vi "Main.vi"() -> ()   [LabVIEW 2020, in "MVA Message Mapper.lvlib"]
doc: "This template is for the Queued Message Handler design pattern.\n\nThe Event Handling Loop generates messages based on user interface actions.\n\nThe Message Handling Loop processes messages generated by the Event Handling Loop, or by other messages. The messages are string values, so new messages can be added easily to the Message Cases case structure in the Message Handling Loop. Each message cluster can also provide an optional value for Message Data, which is a variant that can be converted to whatever message-specific data is required."
uses:
  <vilib>/gpm_packages/@cs/Bus-message-mapper/Source/MVA Message Mapper.lvlib
  <vilib>/gpm_packages/@cs/Bus-message-mapper/Source/controls/UI Data.ctl
  <vilib>/gpm_packages/@cs/Bus-message-mapper/Source/controls/Message Map.ctl
  <vilib>/gpm_packages/@cs/Bus-message-mapper/Source/controls/Map Key.ctl
  <vilib>/gpm_packages/@cs/Bus-message-mapper/Source/controls/Datum Endpoint Set.ctl
  <vilib>/gpm_packages/@cs/Bus-message-mapper/Source/controls/Datum Endpoint.ctl
  <vilib>/gpm_packages/@cs/Bus-message-mapper/Source/support/MVA Comms/MVA Comms VI Instance.lvclass
  <vilib>/gpm_packages/@cs/Bus-message-mapper/Source/support/Format Into String Test/Format Into String.lvclass
  C:/Program Files/National Instruments/LabVIEW 2020/vi.lib/gpm_packages/@cs/Bus-message-mapper/Source/support/Traversal Algorithm/Node Test.lvclass
  <vilib>/gpm_packages/@cs/Bus-message-mapper/Source/support/Build Array Test/Build Array.lvclass
  <vilib>/Utility/miscctls.llb/LVMapReplaceAction.ctl
  <vilib>/gpm_packages/@cs/Bus-message-mapper/Source/support/MVA Comms/MVA Comms VI Instance.lvclass/MVA Comms VI Instance.ctl
  <vilib>/gpm_packages/@cs/Bus-message-mapper/Source/support/MVA Comms/Accessors/Read Broadcaster.vi
  <vilib>/gpm_packages/@cs/Bus-message-mapper/Source/support/Message Queue/Enqueue Message (Single).vi
  <vilib>/Utility/error.llb/Error Cluster From Error Code.vi
  <vilib>/ErrorRing/Error Ring.xnode
panel:
  in  "Load Cache":bool
  out "Refresh Progress":u32(slide) scale=-1.0..37.0
  in  "Cancel Generate":bool
  in  "Generate Cache":bool
  in  "Exit":bool
  in  "Tab Control":enum32{"Message View", "Actor View"}(tab)
  in  "Messages":i32(listbox)=-1
  in  "Broadcasters":i32(listbox)=-1
  in  "Receivers":i32(listbox)=-1
  in  "Actor's Receivers":i32(listbox)=-1
  in  "Actor's Broadcasters":i32(listbox)=-1
  in  "Actor List":i32(listbox)=-1
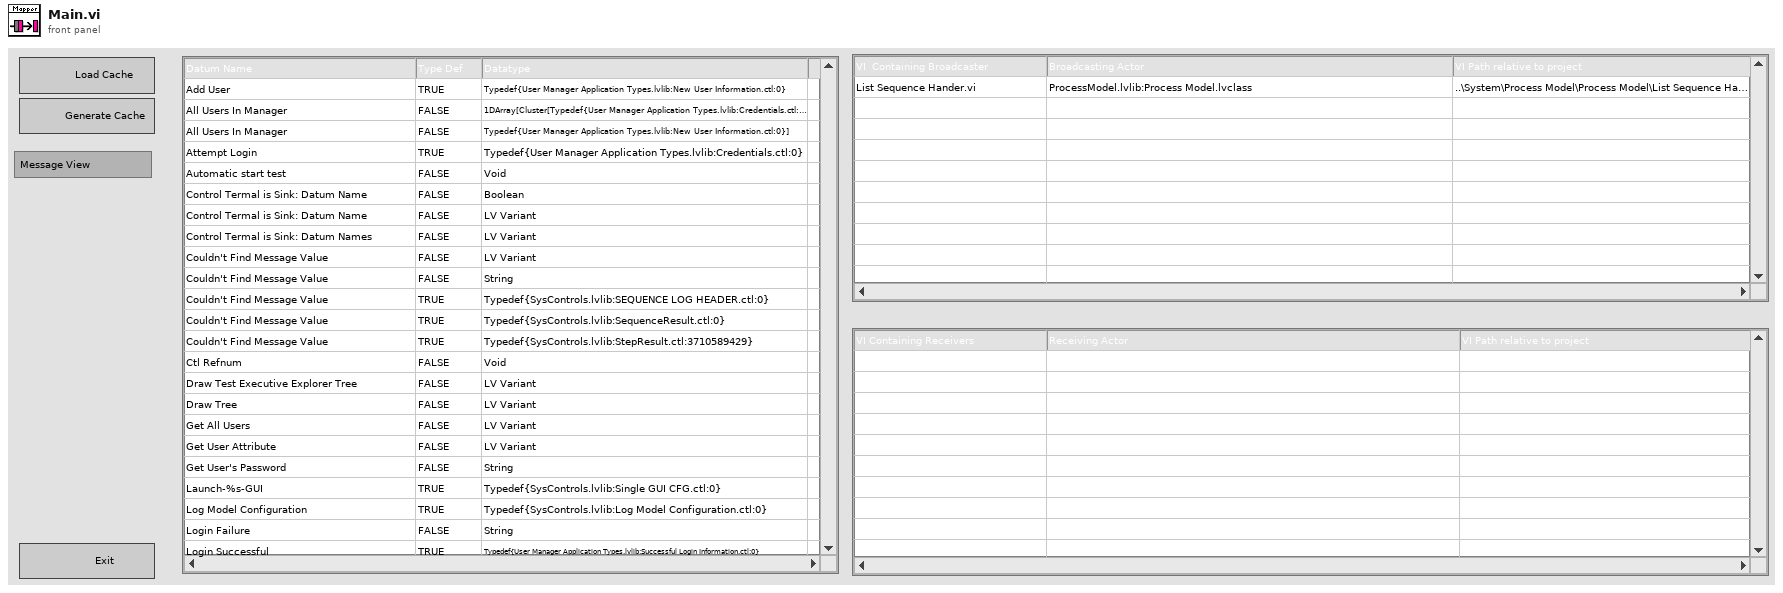
[diagram p1: front panel]
types:
  T1 = typedef "MVA Message Mapper.lvlib/UI Data.ctl" = cluster{"MVA Project Reference":refnum<vi>, "MVA Project Path":path, "Target SubVi Refs":refnum<vi>[], "Targe VI Name":string, "Message View Map":T2, "Broadcaster":bool, "Datum Name Terminal":i32, "Datum Value Terminal":i32, "UI references":cluster{"Message List":refnum<vi>, "Broadcasters":refnum<vi>, "Receivers":refnum<vi>, "Exit Button Ref":refnum<vi>, "Cache Generation Progress":refnum<vi>, "Canced Refresh":refnum<vi>, "Generate Cache":refnum<vi>, "Front Panel":refnum<vi>, "Actor View Receivers":refnum<vi>, "Actor View Broadcasters":refnum<vi>, "Actor View List":refnum<vi>}, "Message Mapper Cache File":path, "MVA Coms VI Instances":refnum<class "MVA Comms VI Instance.lvclass">[], "Cache Generation Marker":u32, "Number of instances":u32, "This VI":refnum<vi>, "Message Map Keys":T3[], "Actor View Map":map{string, cluster{"Datum Broadcasters":T4, "Datum Receivers":T4}}}
  T2 = typedef "MVA Message Mapper.lvlib/Message Map.ctl" = map{T3, cluster{"Datum Broadcasters":T4, "Datum Receivers":T4}}
  T3 = typedef "MVA Message Mapper.lvlib/Map Key.ctl" = cluster{"Datum Name":string, "Value is TypeDef":bool, "Type String":string}
  T4 = typedef "MVA Message Mapper.lvlib/Datum Endpoint Set.ctl" = set{T5}
  T5 = typedef "MVA Message Mapper.lvlib/Datum Endpoint.ctl" = cluster{"Callng VI":path, "Bus VI Name":string, "Source UID":i32, "Sink UID":i32, "Owning Class":string, "Datum Info":T3}
  T6 = typedef "MVA Message Mapper.lvlib/All Message Queues.ctl" = cluster{"UI":refnum<queue>}
  T7 = typedef "LVMapReplaceAction.ctl" = enum32{"Modify Entry only if found", "Add or Modify Entry", "Delete Entry"}
  T8 = enum16{"open", "replace", "create", "open or create", "replace or create", "replace or create with confirmation"}
  T9 = cluster{"VI Name":string, "Owning Actor":string, "Sink UID":string, "Source UID":string}
  T10 = enum32{"Invalid", "Standard", "Closed", "Hidden", "Minimized", "Maximized"}
  T11 = cluster{"Datum Broadcasters":T4, "Datum Receivers":T4}
  T12 = map{string, cluster{"Broadcasters":T4, "Receivers":T4}}
  T13 = map{string, cluster{"Datum Broadcasters":T4, "Datum Receivers":T4}}
  T14 = typedef "LVPoint32TypeDef.ctl" = cluster{"Horizontal":i32, "Vertical":i32}
  T15 = typedef "LVRowAndColumnTypeDef.ctl" = cluster{"Row":i32, "Column":i32}
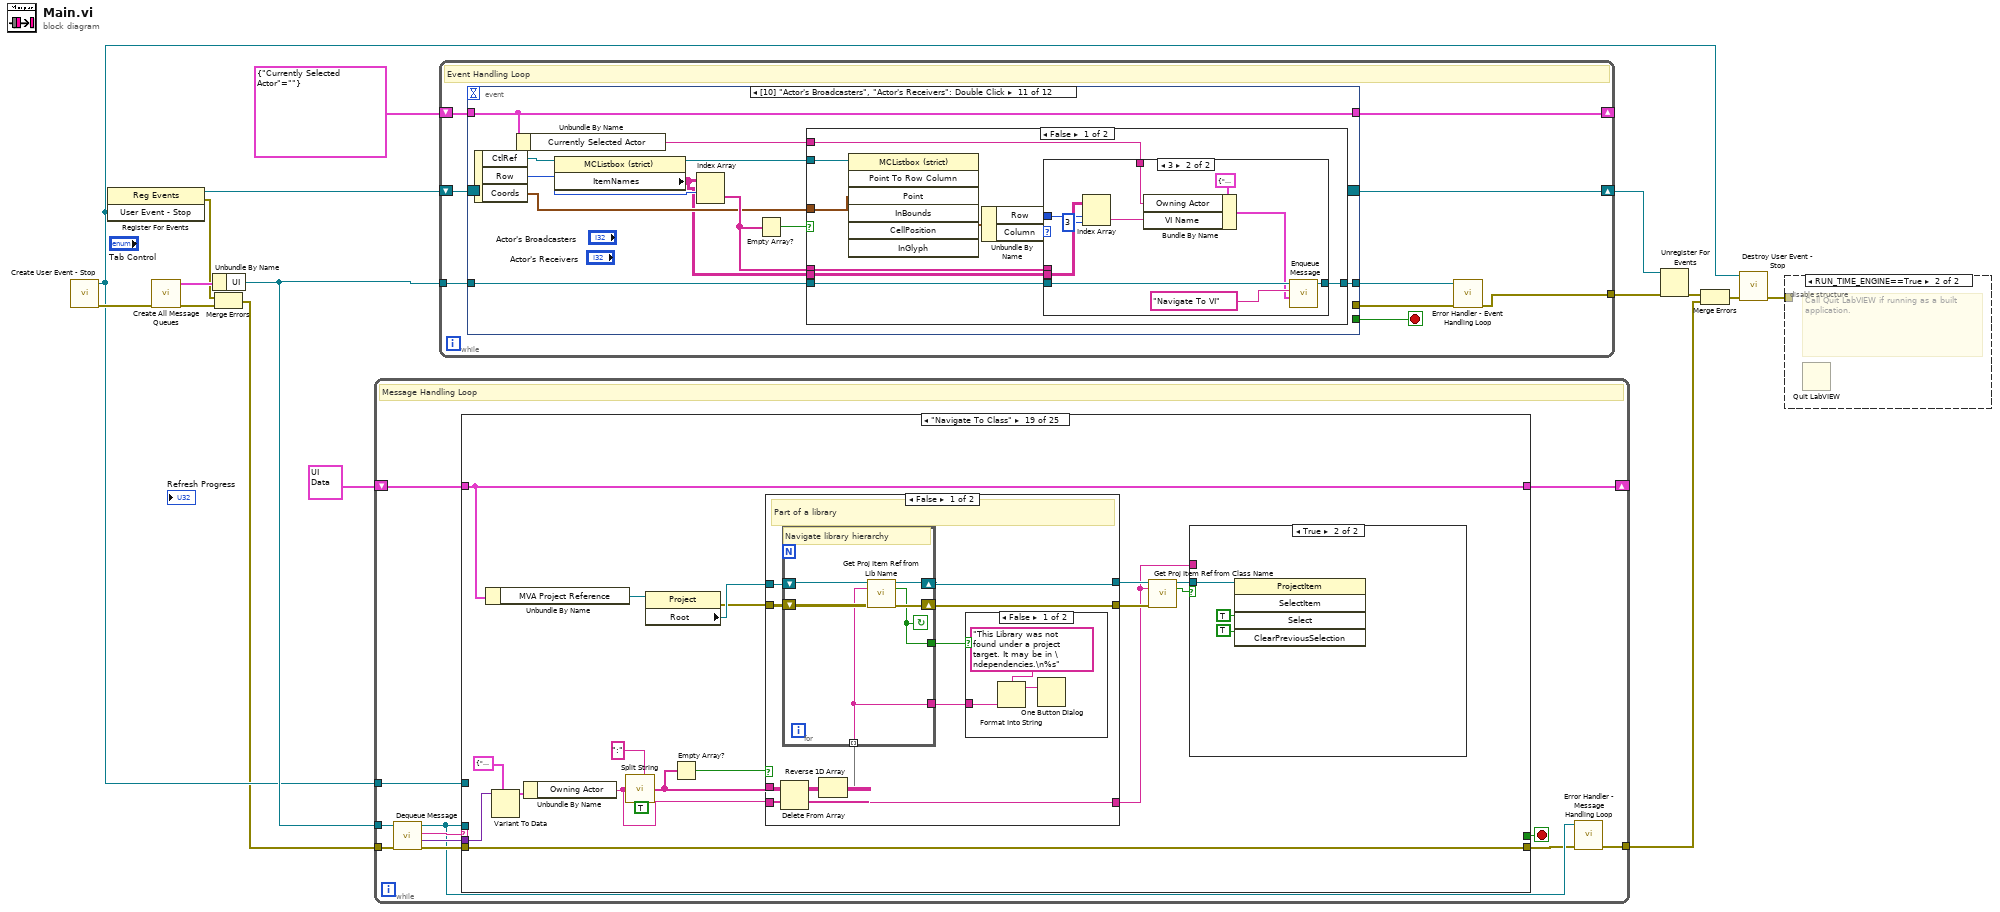
[diagram p0: block diagram]
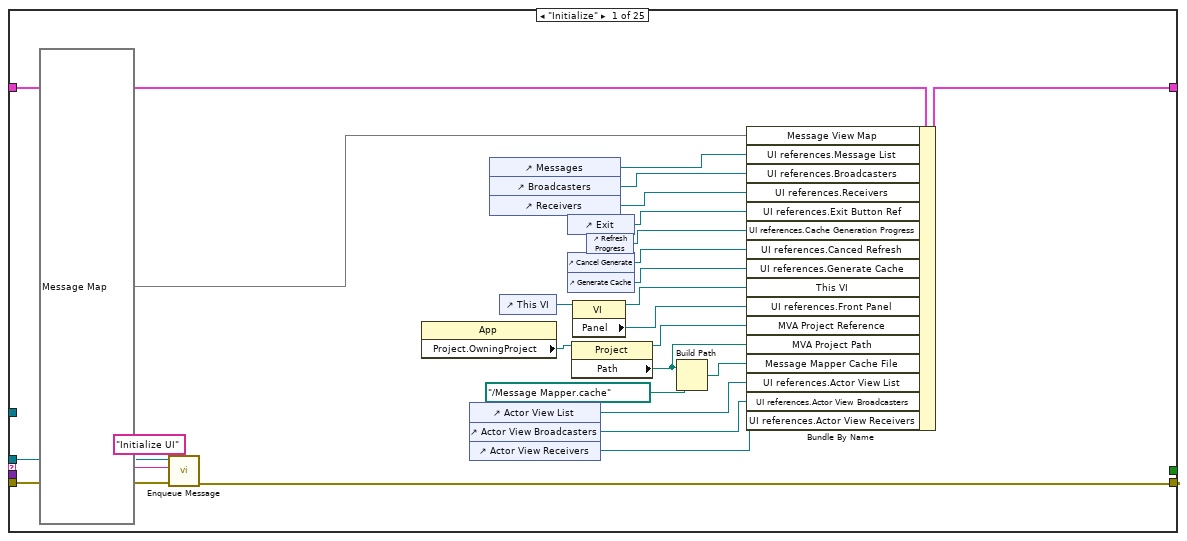
[diagram p2: hidden frame]
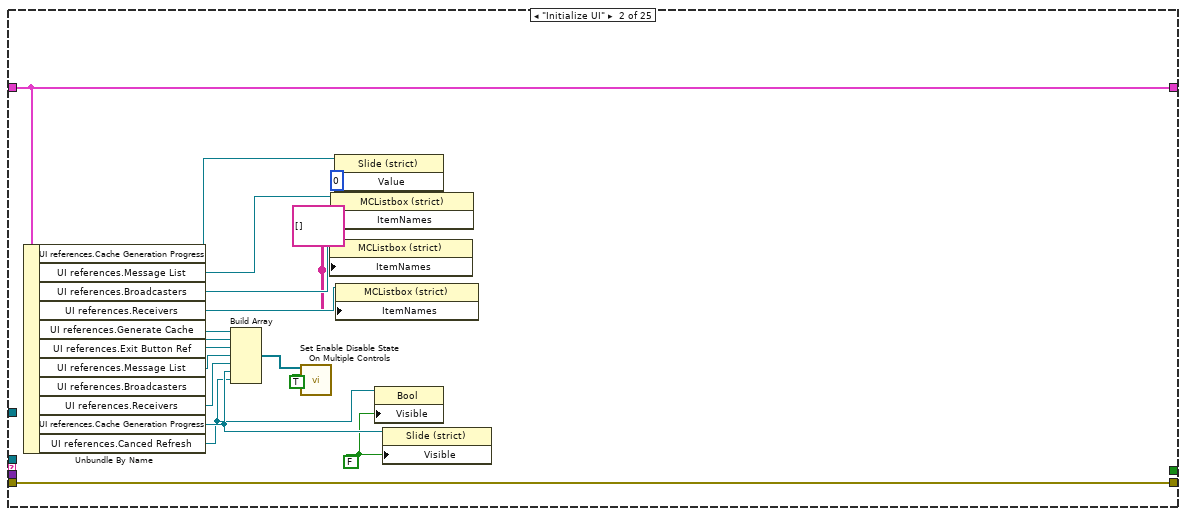
[diagram p3: hidden frame]
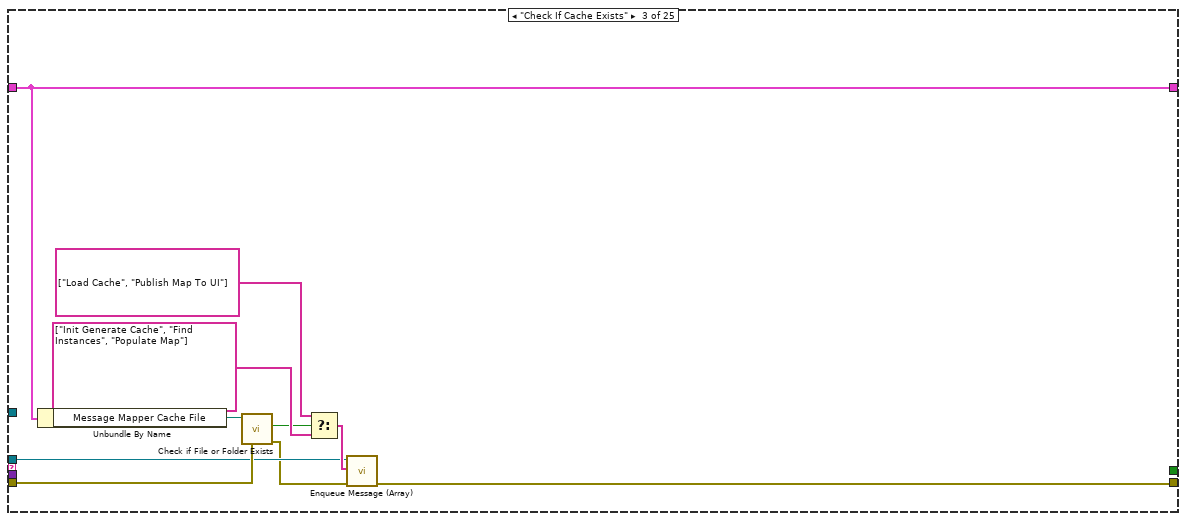
[diagram p4: hidden frame]
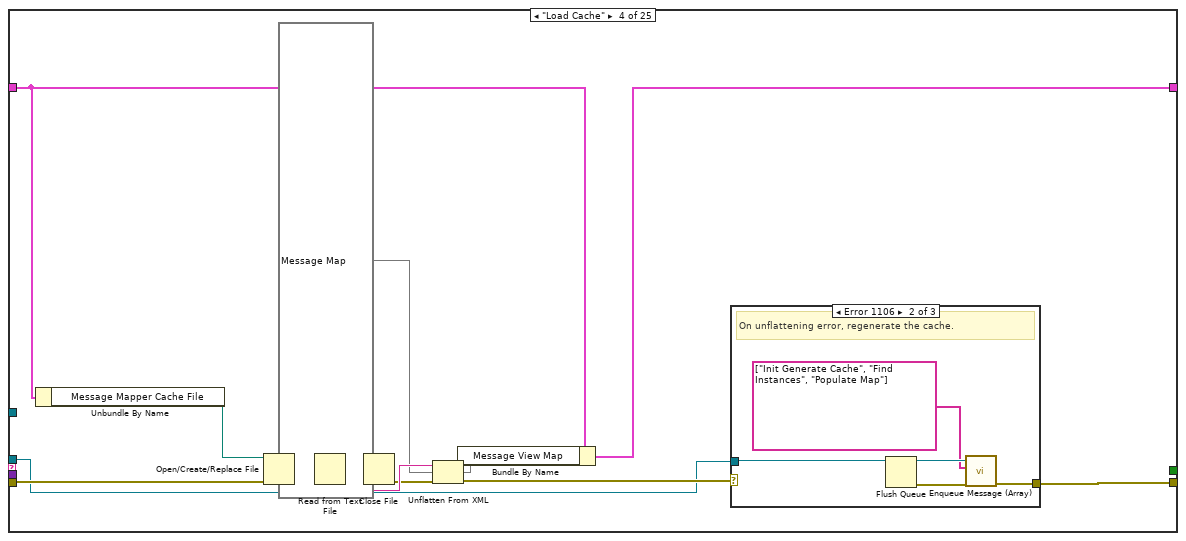
[diagram p5: hidden frame]
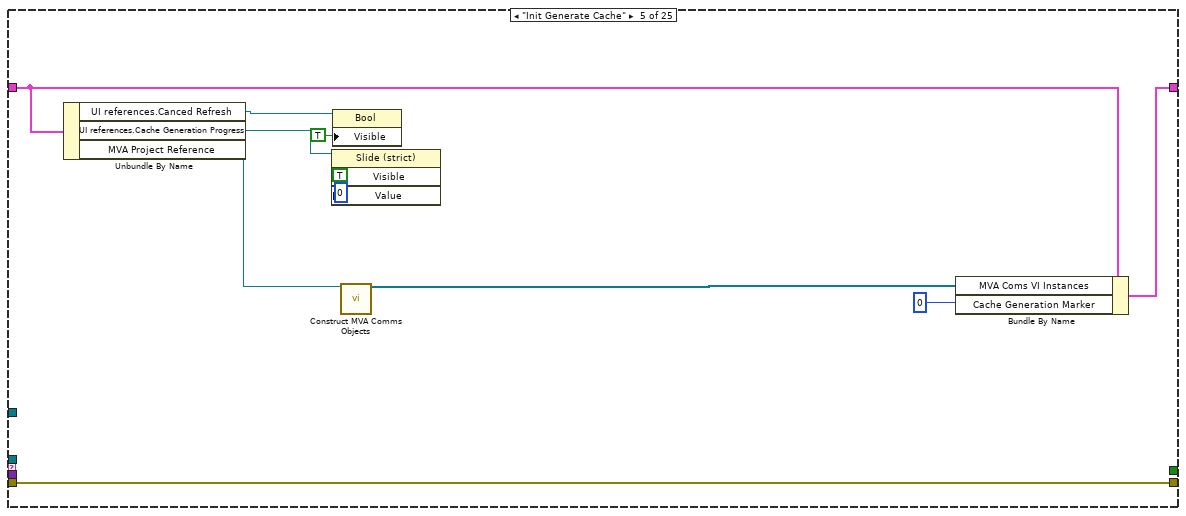
[diagram p8: hidden frame]
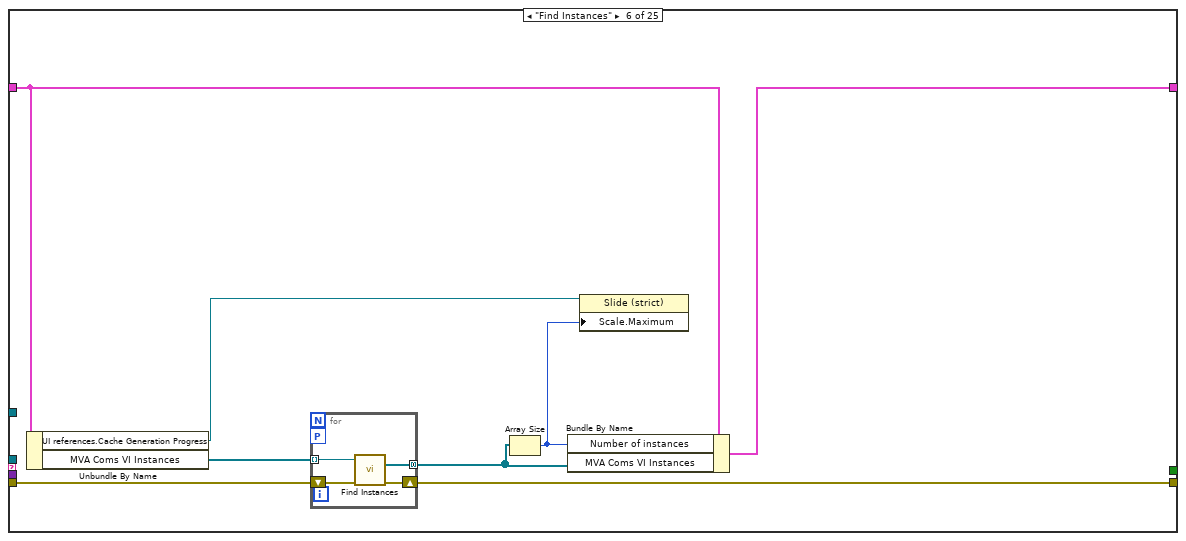
[diagram p9: hidden frame]
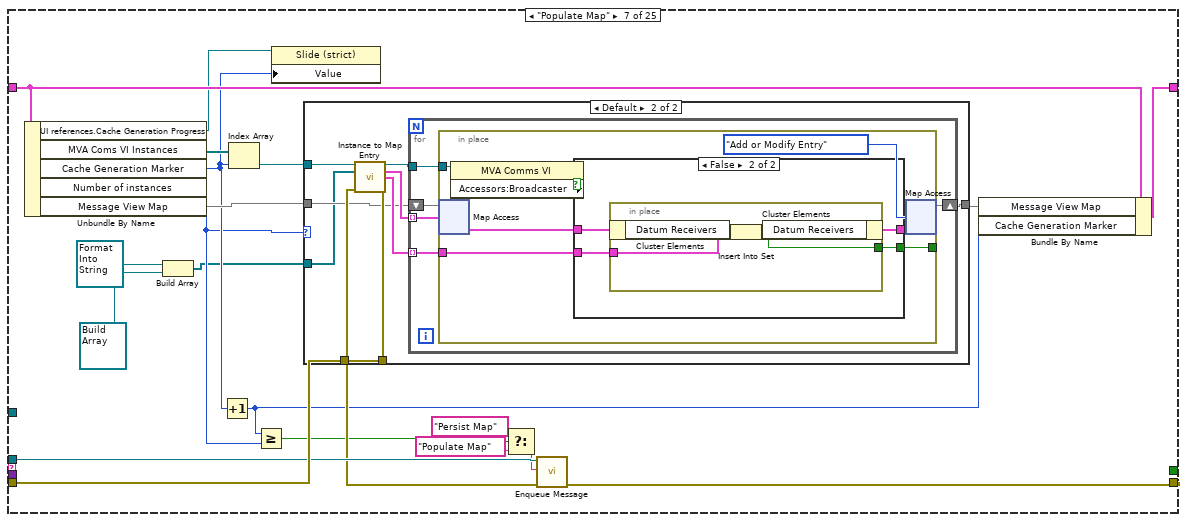
[diagram p10: hidden frame]
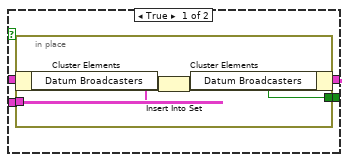
[diagram p12: hidden frame]
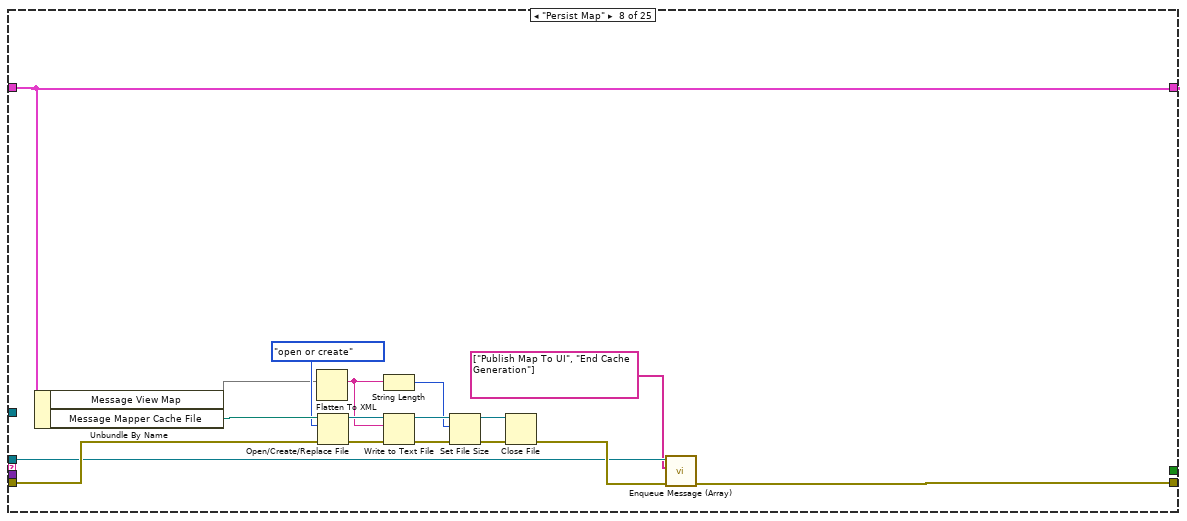
[diagram p13: hidden frame]
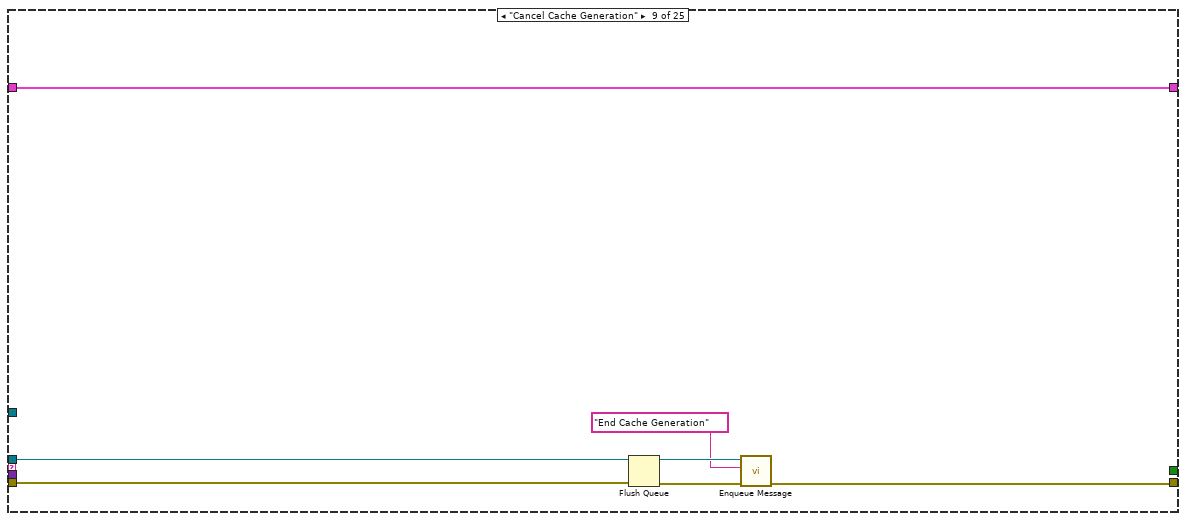
[diagram p14: hidden frame]
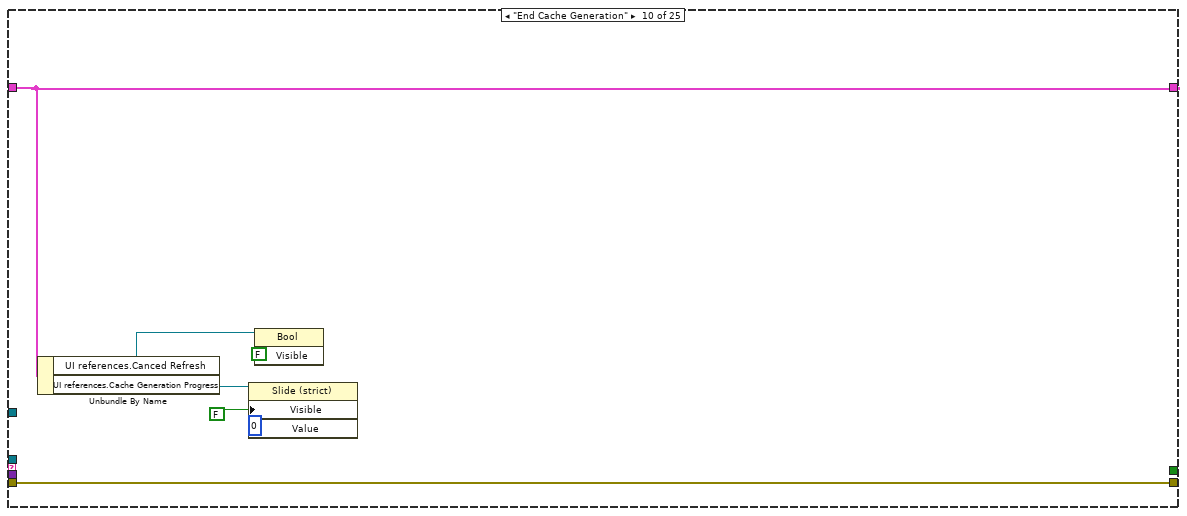
[diagram p15: hidden frame]
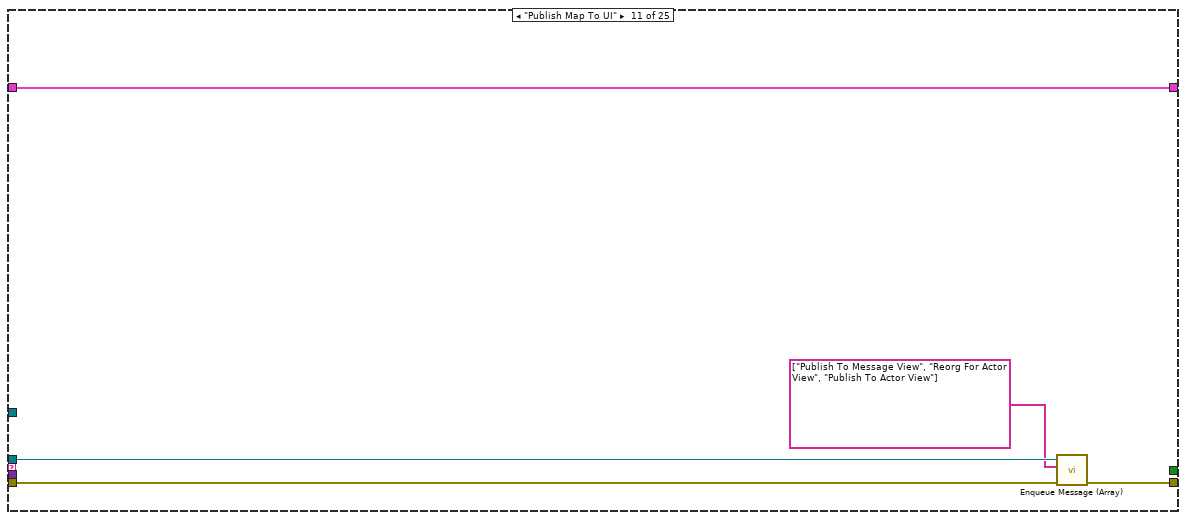
[diagram p16: hidden frame]
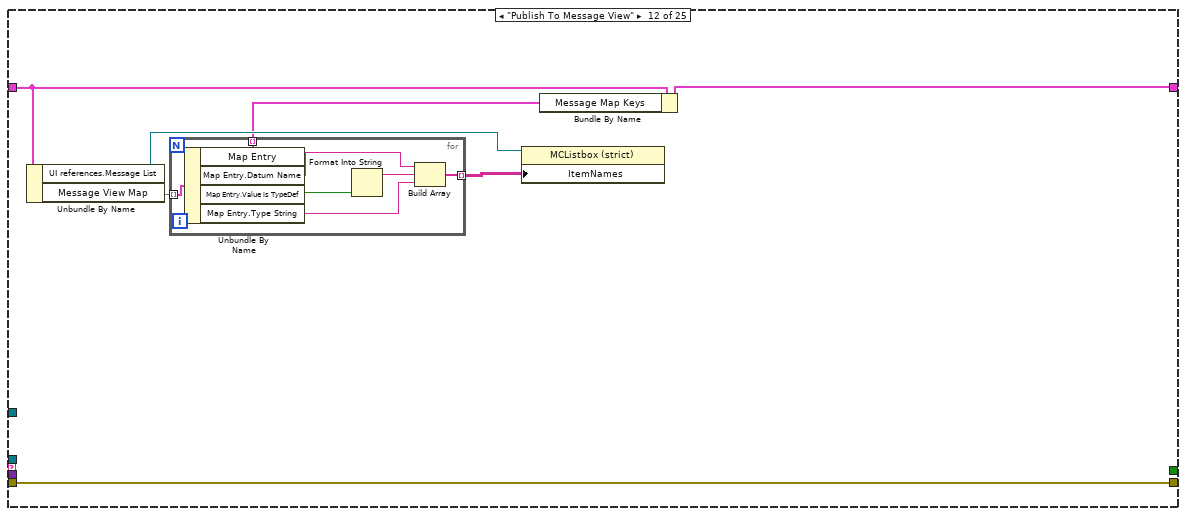
[diagram p17: hidden frame]
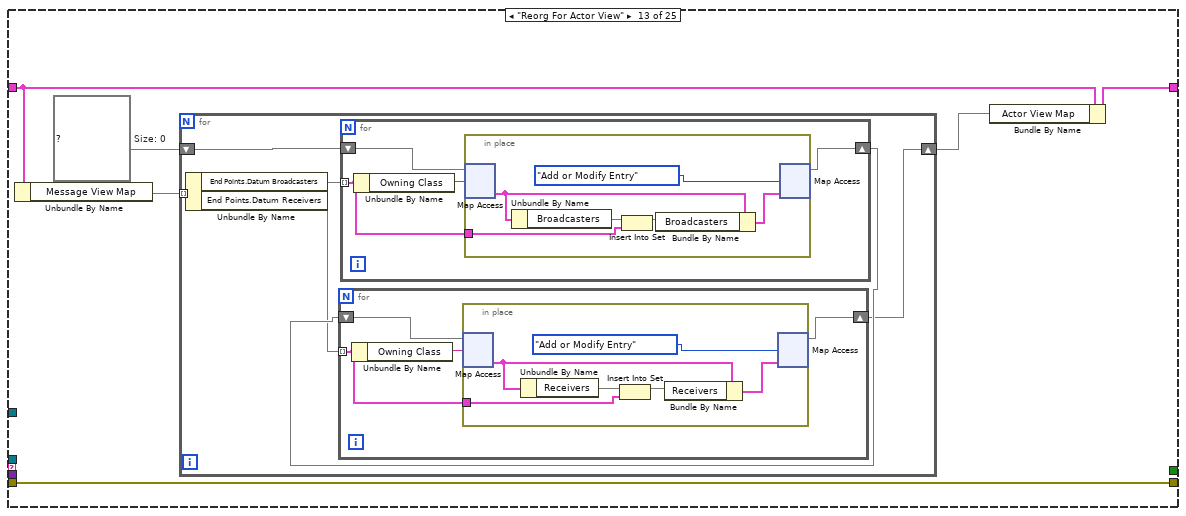
[diagram p18: hidden frame]
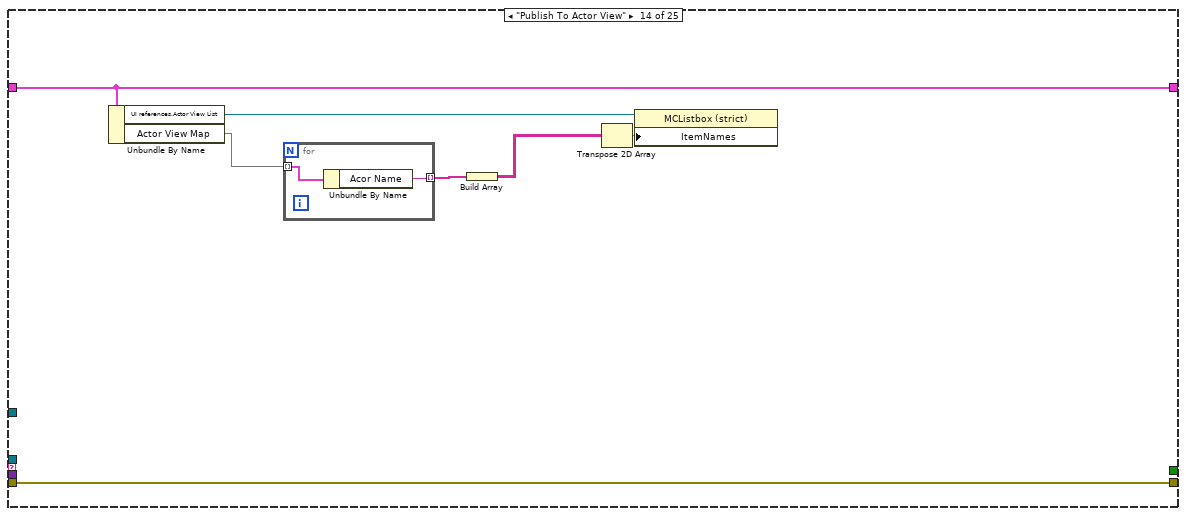
[diagram p19: hidden frame]
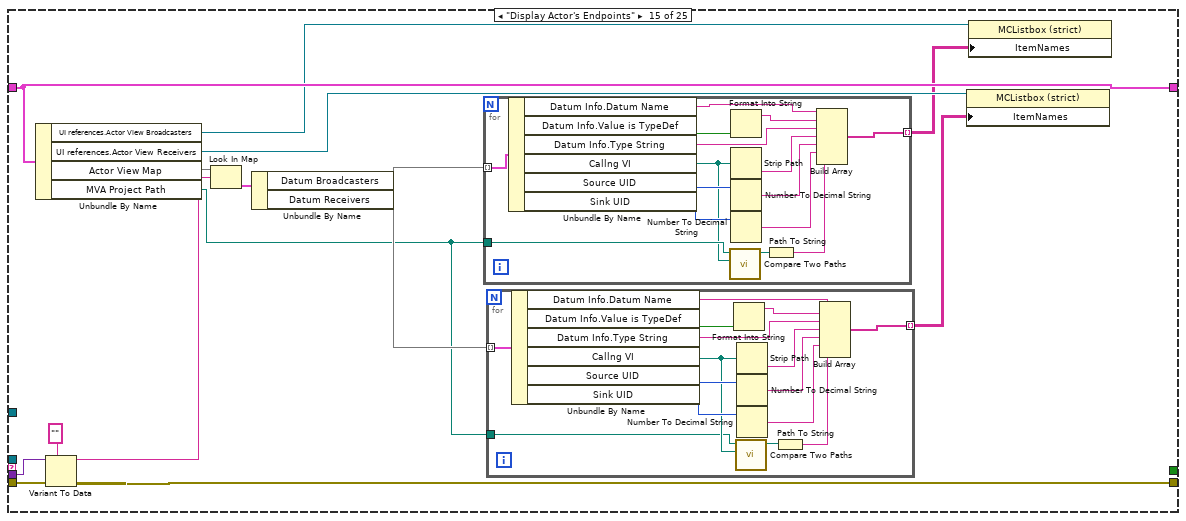
[diagram p20: hidden frame]
diagram:
  n1 = call <vilib>:"Create User Event - Stop.vi"() -> ("error out"=w12:errorcluster, "User Event - Stop"=w4:refnum<user-event>)  [unwired: 10 in]
  n2 = register-events(w4) -> (reference out=w5:refnum<event-registration>, error out=w2:errorcluster)  [unwired: 2 in]
  n3 = call <vilib>:"Create All Message Queues.vi"("error in (no error)"=w12) -> ("error out"=w16:errorcluster, "Message Queues out"=w15:T6)  [unwired: 9 in]
  n4 = Unbundle By Name(w15) -> ("UI"=w13:refnum<queue>)
  n5 = Merge Errors(w2, w16) -> (w3:errorcluster)
  n6 = while {
    tunnel: w13 -> [w20]
    shift-right: [w27] -> _
    shift-left: T1 {"MVA Project Reference"=refnum, "MVA Project Path"=path "", "Target SubVi Refs"=[], "Targe VI Name"="", "Message View Map"={}, "Broadcaster"=FALSE, "Datum Name Terminal"=0, "Datum Value Terminal"=0, "UI references"={"Message List"=refnum, "Broadcasters"=refnum, "Receivers"=refnum, "Exit Button Ref"=refnum, "Cache Generation Progress"=refnum, "Canced Refresh"=refnum, "Generate Cache"=refnum, "Front Panel"=refnum, "Actor View Receivers"=refnum, "Actor View Broadcasters"=refnum, "Actor View List"=refnum}, "Message Mapper Cache File"=path "", "MVA Coms VI Instances"=[], "Cache Generation Marker"=0, "Number of instances"=0, "This VI"=refnum, "Message Map Keys"=[], "Actor View Map"={}} ("Data Cluster") -> [w28]
    tunnel: w4 -> [w25]
    tunnel: w3 -> [w24]
    tunnel: [w18] -> w14
    stop <- w26 stop-if-true
    # "Message Handling Loop"
    n7 = call <vilib>:"Dequeue Message.vi"("error in (no error)"=w24, "Message Queue"=w20) -> ("error out"=w23:errorcluster, "Message Data"=w21:variant, "Message"=w22:string, "dup Message Queue"=w19:refnum<queue>)  [unwired: 6 in]
    n8 = case "Message Cases" shown="\"Navigate To Class\"" w22 {
      selector: w22 -> [_ _ _ _ _ _ _ _ _ _ _ _ _ _ _ _ _ _ _ _ _ _ _ _ w570]
      tunnel: w19 -> [w49 _ w73 w83 _ _ w141 w189 w209 _ w219 _ _ _ _ _ _ _ _ _ _ w551 _ w569 _]
      tunnel: w23 -> [w52 w71 w80 w94 w105 w121 w143 w194 w208 w216 w221 w223 w239 w275 w291 w339 w384 w456 w507 w539 w548 w555 w558 w562 _]
      tunnel: [w53 w71 w78 w82 w105 w119 w139 w188 w205 w216 w220 w223 w239 w275 w290 w338 w382 w456 w507 w540 w542 w553 w556 w565 w571] -> w17
      tunnel: w28 -> [w39 w70 w81 w96 w114 w122 w147 w203 w210 w217 w222 w227 w241 w274 w288 w335 w383 w446 w505 w541 w547 w554 w557 w568 w572]
      tunnel: [w51 w70 w81 w87 w113 w120 w144 w203 w210 w217 w222 w225 w238 w274 w288 w335 w383 w446 w505 w541 w547 w554 w557 w568 w572] -> w27
      tunnel: [_ _ _ _ _ _ _ _ _ _ _ _ _ _ _ _ _ _ _ _ _ _ _ TRUE _] -> w26
      tunnel: w21 -> [_ _ _ _ _ _ _ _ _ _ _ _ _ _ w292 w337 w385 w455 w506 w538 w546 _ _ w559 _]
      tunnel: w25 -> [_ _ _ _ _ _ _ _ _ _ _ _ _ _ _ _ _ _ _ _ _ _ _ w564 _]
      frame "Initialize" {
        # "Initialize - All initialization work should take place in this message, since other loops can potentially enqueue messages that execute immediately after this one."
        n9 = call-poly <vilib>:"Enqueue Message.vi"("error in (no error)"=w52, "Message"="Initialize UI", "Message Queue"=w49) -> ("error out"=w53:errorcluster)  [unwired: 7 in, 1 out]
        n10 = property class="App"() -> ("Project.OwningProject"=w36:refnum<vi>)  [unwired: 2 in, 2 out]
        n11 = control-ref of="Actor View List"() -> (w31:refnum<vi>)
        n12 = control-ref of="Actor View Broadcasters"() -> (w30:refnum<vi>)
        n13 = control-ref of="Actor View Receivers"() -> (w29:refnum<vi>)
        n14 = control-ref of="Messages"() -> (w42:refnum<vi>)
        n15 = control-ref of="Broadcasters"() -> (w43:refnum<vi>)
        n16 = control-ref of="Receivers"() -> (w44:refnum<vi>)
        n17 = control-ref of="This VI"() -> (w41:refnum<vi>)
        n18 = control-ref of="Exit"() -> (w45:refnum<vi>)
        n19 = control-ref of="Cancel Generate"() -> (w47:refnum<vi>)
        n20 = control-ref of="Generate Cache"() -> (w46:refnum<vi>)
        n21 = property class="Project"(reference=w36) -> (reference out=w33:refnum<vi>, "Path"=w34:path)  [unwired: 1 in, 1 out]
        n22 = property class="VI"(reference=w41) -> (reference out=w37:refnum<vi>, "Panel"=w40:refnum<vi>)  [unwired: 1 in, 1 out]
        n23 = control-ref of="Refresh Progress"() -> (w48:refnum<vi>)
        n24 = Build Path(base path=w34, name or relative path=path "../Message Mapper.cache") -> (appended path=w32:path)
        n25 = Bundle By Name(cluster=w39, "Message View Map"=T2 {} ("Message Map"), "UI references.Message List"=w42, "UI references.Broadcasters"=w43, "UI references.Receivers"=w44, "UI references.Exit Button Ref"=w45, "UI references.Cache Generation Progress"=w48, "UI references.Canced Refresh"=w47, "UI references.Generate Cache"=w46, "This VI"=w37, "UI references.Front Panel"=w40, "MVA Project Reference"=w33, "MVA Project Path"=w34, "Message Mapper Cache File"=w32, "UI references.Actor View List"=w31, "UI references.Actor View Broadcasters"=w30, "UI references.Actor View Receivers"=w29) -> (w51:T1)
      }
      frame "Initialize UI" {
        w56 = string[][] [] ("Item Names")
        w60 = FALSE
        n26 = Unbundle By Name(w70) -> ("UI references.Cache Generation Progress"=w55:refnum<vi>, "UI references.Message List"=w59:refnum<vi>, "UI references.Broadcasters"=w58:refnum<vi>, "UI references.Receivers"=w57:refnum<vi>, "UI references.Generate Cache"=w65:refnum<vi>, "UI references.Exit Button Ref"=w69:refnum<vi>, "UI references.Message List"=w64:refnum<vi>, "UI references.Broadcasters"=w63:refnum<vi>, "UI references.Receivers"=w62:refnum<vi>, "UI references.Cache Generation Progress"=w66:refnum<vi>, "UI references.Canced Refresh"=w61:refnum<vi>)
        n27 = Build Array(w65, w69, w64, w63, w62, w66, w61) -> (w68:refnum<vi>[])
        n28 = call <vilib>:"Set Enable Disable State On Multiple Controls.vi"("Controls"=w68, "Enable?"=TRUE) -> ()  [unwired: 14 in]
        n29 = property class="MCListbox (strict)"(reference=w58, "ItemNames"=w56) -> ()  [unwired: 1 in, 2 out]
        n30 = property class="MCListbox (strict)"(reference=w59, "ItemNames"=w56) -> ()  [unwired: 1 in, 2 out]
        n31 = property class="Slide (strict)"(reference=w55, "Value"=u32 0) -> ()  [unwired: 1 in, 2 out]
        n32 = property class="MCListbox (strict)"(reference=w57, "ItemNames"=w56) -> ()  [unwired: 1 in, 2 out]
        n33 = property class="Bool"(reference=w61, "Visible"=w60) -> ()  [unwired: 1 in, 2 out]
        n34 = property class="Slide (strict)"(reference=w66, "Visible"=w60) -> ()  [unwired: 1 in, 2 out]
      }
      frame "Check If Cache Exists" {
        n35 = Unbundle By Name(w81) -> ("Message Mapper Cache File"=w79:path)
        n36 = call <vilib>:"Check if File or Folder Exists.vi"("error in (no error)"=w80, "path"=w79) -> ("error out"=w72:errorcluster, "file or folder exists?"=w75:bool)  [unwired: 7 in, 1 out]
        n37 = Select(t=string[] ["Load Cache", "Publish Map To UI"] ("Message Array"), s=w75, f=string[] ["Init Generate Cache", "Find Instances", "Populate Map"] ("Message Array")) -> (s? t:f=w74:string[])
        n38 = call <vilib>:"Enqueue Message (Array).vi"("error in (no error)"=w72, "Message Array"=w74, "Message Queue"=w73) -> ("error out"=w78:errorcluster)  [unwired: 7 in, 1 out]
      }
      frame "Load Cache" {
        n39 = Unbundle By Name(w96) -> ("Message Mapper Cache File"=w95:path)
        n40 = Open/Create/Replace File(file path (use dialog)=w95, error in=w94) -> (refnum out=w92:refnum<file>, error out=w93:errorcluster)  [unwired: 4 in, 1 out]
        n41 = Read from Text File(file (use dialog)=w92, error in=w93) -> (refnum out=w91:refnum<file>, text=w89:string, error out=w90:errorcluster)  [unwired: 2 in, 1 out]
        n42 = Close File(refnum=w91, error in=w90) -> (error out=w85:errorcluster)  [unwired: 1 out]
        n43 = Unflatten From XML(xml string=w89, type=T2 {} ("Message Map"), error in (no error)=w85) -> (value=w86:T2, error out=w84:errorcluster)
        n44 = Bundle By Name(cluster=w96, "Message View Map"=w86) -> (w87:T1)
        n45 = case shown="Error 1106" w84 {
          selector: w84 -> [w97 _ w103]
          tunnel: w83 -> [_ w102 _]
          tunnel: [w97 w98 w103] -> w82
          frame No Error {
          }
          frame Error {
            # "On unflattening error, regenerate the cache."
            n46 = Flush Queue(queue=w102) -> (queue out=w101:refnum<queue>, error out=w99:errorcluster)  [unwired: 1 in, 1 out]
            n47 = call <vilib>:"Enqueue Message (Array).vi"("error in (no error)"=w99, "Message Array"=string[] ["Init Generate Cache", "Find Instances", "Populate Map"], "Message Queue"=w101) -> ("error out"=w98:errorcluster)  [unwired: 7 in, 1 out]
          }
          frame Default {
          }
        }
      }
      frame "Init Generate Cache" {
        n48 = Unbundle By Name(w114) -> ("UI references.Canced Refresh"=w107:refnum<vi>, "UI references.Cache Generation Progress"=w111:refnum<vi>, "MVA Project Reference"=w106:refnum<vi>)
        n49 = property class="Slide (strict)"(reference=w111, "Visible"=TRUE, "Value"=u8 0) -> ()  [unwired: 1 in, 2 out]
        n50 = property class="Bool"(reference=w107, "Visible"=TRUE) -> ()  [unwired: 1 in, 2 out]
        n51 = call <vilib>:"Construct MVA Comms Objects.vi"("MVA Project Reference"=w106) -> ("MVA Comms VIs"=w104:refnum<class "MVA Comms VI Instance.lvclass">[])  [unwired: 14 in]
        n52 = Bundle By Name(cluster=w114, "MVA Coms VI Instances"=w104, "Cache Generation Marker"=u32 0) -> (w113:T1)
      }
      frame "Find Instances" {
        n53 = Unbundle By Name(w122) -> ("UI references.Cache Generation Progress"=w117:refnum<vi>, "MVA Coms VI Instances"=w115:refnum<class "MVA Comms VI Instance.lvclass">[])
        n54 = for {
          tunnel: w115 -> [w126] mode=indexing
          tunnel: [w125] -> w118 mode=concatenating
          shift-right: [w123] -> w119
          shift-left: w121 -> [w124]
          workers-P: _ -> [_]
          n55 = call-dynamic "Find Instances.vi"("MVA Comms VI in"=w126, "error in (no error)"=w124) -> ("Instances"=w125:refnum<class "MVA Comms VI Instance.lvclass">[], "error out"=w123:errorcluster)  [unwired: 11 in, 1 out]
        }
        n56 = Array Size(array=w118) -> (size(s)=w116:i32)
        n57 = Bundle By Name(cluster=w122, "Number of instances"=w116, "MVA Coms VI Instances"=w118) -> (w120:T1)
        n58 = property class="Slide (strict)"(reference=w117, "Scale.Maximum"=w116) -> ()  [unwired: 1 in, 2 out]
      }
      frame "Populate Map" {
        n59 = Unbundle By Name(w147) -> ("UI references.Cache Generation Progress"=w132:refnum<vi>, "MVA Coms VI Instances"=w146:refnum<class "MVA Comms VI Instance.lvclass">[], "Cache Generation Marker"=w131:u32, "Number of instances"=w130:u32, "Message View Map"=w135:T2)
        n60 = Build Array(refnum<class "Format Into String.lvclass"> refnum ("MVA Message Mapper.lvlib:Format Into String.lvclass"), refnum<class "Build Array.lvclass"> refnum ("MVA Message Mapper.lvlib:Build Array.lvclass")) -> (w129:refnum<class "Node Test.lvclass">[])
        n61 = Increment(x=w131) -> (x+1=w133:u32)
        n62 = Index Array(array=w146, index=w131) -> (element=w145:refnum<class "MVA Comms VI Instance.lvclass">)
        n63 = Greater Or Equal?(x=w133, y=w130) -> (x >= y?=w138:bool)
        n64 = property class="Slide (strict)"(reference=w132, "Value"=w131) -> ()  [unwired: 1 in, 2 out]
        n65 = case shown="Default" w130 {
          tunnel: w145 -> [_ w158]
          tunnel: w143 -> [w148 w156]
          tunnel: [w149 w153] -> w142
          tunnel: [w148 w152] -> w140
          tunnel: w135 -> [w149 w151]
          tunnel: w129 -> [_ w150]
          frame 0 {
          }
          frame Default {
            n66 = call-dynamic "Instance to Map Entry.vi"("MVA Comms VI in"=w158, "Node Tests"=w150, "error in (no error)"=w156) -> ("MVA Comms VI out"=w154:refnum<class "MVA Comms VI Instance.lvclass">, "Map Key"=w157:T3[], "Array"=w155:T5[], "error out"=w152:errorcluster)  [unwired: 9 in]
            n67 = for {
              tunnel: w157 -> [w163] mode=indexing
              tunnel: w155 -> [w162] mode=indexing
              tunnel: w154 -> [w161]
              shift-right: [w160] -> w153
              shift-left: w151 -> [w159]
              n68 = in-place {
                in-place-border: w162 -> [w167]
                in-place-border: w161 -> [w166]
                in-place-border: [w164] -> _
                n69 = in-place-map #1(w159, w163) -> (w170:T11)  [unwired: 1 in, 1 out]
                n70 = property class="MVA Comms VI"(reference=w166) -> ("Accessors:Broadcaster"=w165:bool)  [unwired: 1 in, 2 out]
                n71 = case shown="False" w165 {
                  tunnel: w170 -> [w174 w182]
                  tunnel: [w173 w181] -> w169
                  tunnel: w167 -> [w172 w180]
                  tunnel: [w171 w179] -> w164
                  frame True {
                    n72 = in-place {
                      in-place-border: w172 -> [w176]
                      in-place-border: [w175] -> w171
                      n73 = in-place-cluster #2(w174) -> ("Datum Broadcasters"=w178:T4)
                      n74 = Insert Into Set(10:w176, 11:w178) -> (2:w175:bool, 3:w177:T4)
                      n75 = in-place-cluster #2("Datum Broadcasters"=w177) -> (w173:T11)
                    }
                  }
                  frame False {
                    n76 = in-place {
                      in-place-border: w180 -> [w184]
                      in-place-border: [w183] -> w179
                      n77 = in-place-cluster #3(w182) -> ("Datum Receivers"=w185:T4)
                      n78 = Insert Into Set(10:w184, 11:w185) -> (2:w183:bool, 3:w186:T4)
                      n79 = in-place-cluster #3("Datum Receivers"=w186) -> (w181:T11)
                    }
                  }
                }
                n80 = in-place-map #1(w169, LVMapReplaceAction."Add or Modify Entry" ("action")) -> (w160:T2)  [unwired: 2 out]
              }
            }
          }
        }
        n81 = Select(t="Persist Map" ("Message"), s=w138, f="Populate Map" ("Message")) -> (s? t:f=w137:string)
        n82 = call-poly <vilib>:"Enqueue Message.vi"("error in (no error)"=w140, "Message"=w137, "Message Queue"=w141) -> ("error out"=w139:errorcluster)  [unwired: 7 in, 1 out]
        n83 = Bundle By Name(cluster=w147, "Message View Map"=w142, "Cache Generation Marker"=w133) -> (w144:T1)
      }
      frame "Persist Map" {
        n84 = Unbundle By Name(w203) -> ("Message View Map"=w190:T2, "Message Mapper Cache File"=w202:path)
        n85 = Flatten To XML(6:w190) -> (2:w192:string)
        n86 = Open/Create/Replace File(file path (use dialog)=w202, error in=w194, operation (0:open)=T8."open or create") -> (refnum out=w201:refnum<file>, error out=w196:errorcluster)  [unwired: 3 in, 1 out]
        n87 = String Length(string=w192) -> (length=w191:i32)
        n88 = Write to Text File(file (use dialog)=w201, text=w192, error in=w196) -> (refnum out=w199:refnum<file>, error out=w200:errorcluster)  [unwired: 1 in, 1 out]
        n89 = Set File Size(4:w200, 6:w191, 7:w199) -> (0:w197:errorcluster, 3:w198:refnum<file>)
        n90 = Close File(refnum=w198, error in=w197) -> (error out=w193:errorcluster)  [unwired: 1 out]
        n91 = call <vilib>:"Enqueue Message (Array).vi"("error in (no error)"=w193, "Message Array"=string[] ["Publish Map To UI", "End Cache Generation"], "Message Queue"=w189) -> ("error out"=w188:errorcluster)  [unwired: 7 in, 1 out]
      }
      frame "Cancel Cache Generation" {
        n92 = Flush Queue(queue=w209, error in (no error)=w208) -> (queue out=w207:refnum<queue>, error out=w206:errorcluster)  [unwired: 1 out]
        n93 = call-poly <vilib>:"Enqueue Message.vi"("error in (no error)"=w206, "Message"="End Cache Generation", "Message Queue"=w207) -> ("error out"=w205:errorcluster)  [unwired: 7 in, 1 out]
      }
      frame "End Cache Generation" {
        n94 = Unbundle By Name(w217) -> ("UI references.Canced Refresh"=w212:refnum<vi>, "UI references.Cache Generation Progress"=w215:refnum<vi>)
        n95 = property class="Slide (strict)"(reference=w215, "Visible"=FALSE, "Value"=u8 0) -> ()  [unwired: 1 in, 2 out]
        n96 = property class="Bool"(reference=w212, "Visible"=FALSE) -> ()  [unwired: 1 in, 2 out]
      }
      frame "Publish Map To UI" {
        n97 = call <vilib>:"Enqueue Message (Array).vi"("error in (no error)"=w221, "Message Array"=string[] ["Publish To Message View", "Reorg For Actor View", "Publish To Actor View"], "Message Queue"=w219) -> ("error out"=w220:errorcluster)  [unwired: 7 in, 1 out]
      }
      frame "Publish To Message View" {
        n98 = Unbundle By Name(w227) -> ("UI references.Message List"=w226:refnum<vi>, "Message View Map"=w228:T2)
        n99 = for {
          tunnel: w228 -> [w232] mode=indexing
          tunnel: [w235] -> w229 mode=indexing
          tunnel: [w231] -> w224 mode=indexing
          n100 = Unbundle By Name(w232) -> ("Map Entry"=w231:T3, "Map Entry.Datum Name"=w233:string, "Map Entry.Value is TypeDef"=w236:bool, "Map Entry.Type String"=w230:string)
          n101 = Format Into String(w236) -> (resulting string=w234:string)  [unwired: 3 in, 1 out]
          n102 = Build Array(w233, w234, w230) -> (w235:string[])
        }
        n103 = property class="MCListbox (strict)"(reference=w226, "ItemNames"=w229) -> ()  [unwired: 1 in, 2 out]
        n104 = Bundle By Name(cluster=w227, "Message Map Keys"=w224) -> (w225:T1)
      }
      frame "Reorg For Actor View" {
        w240 = T12 {}  # Size: 0
        n105 = Unbundle By Name(w241) -> ("Message View Map"=w242:T2)
        n106 = for {
          tunnel: w242 -> [w248] mode=indexing
          shift-right: [w243] -> w237
          shift-left: w240 -> [w246]
          n107 = Unbundle By Name(w248) -> ("End Points.Datum Broadcasters"=w247:T4, "End Points.Datum Receivers"=w244:T4)
          n108 = for {
            tunnel: w247 -> [w259] mode=indexing
            shift-right: [w260] -> w245
            shift-left: w246 -> [w261]
            n109 = Unbundle By Name(w259) -> ("Owning Class"=w262:string)
            n110 = in-place {
              in-place-border: w259 -> [w266]
              n111 = in-place-map #4(w261, w262) -> (w265:cluster{"Broadcasters":T4, "Receivers":T4})  [unwired: 1 in, 1 out]
              n112 = Unbundle By Name(w265) -> ("Broadcasters"=w267:T4)
              n113 = Insert Into Set(10:w266, 11:w267) -> (3:w264:T4)  [unwired: 1 out]
              n114 = Bundle By Name(cluster=w265, "Broadcasters"=w264) -> (w263:cluster{"Broadcasters":T4, "Receivers":T4})
              n115 = in-place-map #4(w263, LVMapReplaceAction."Add or Modify Entry" ("action")) -> (w260:T12)  [unwired: 2 out]
            }
          }
          n116 = for {
            tunnel: w244 -> [w249] mode=indexing
            shift-right: [w250] -> w243
            shift-left: w245 -> [w251]
            n117 = Unbundle By Name(w249) -> ("Owning Class"=w252:string)
            n118 = in-place {
              in-place-border: w249 -> [w256]
              n119 = in-place-map #5(w251, w252) -> (w255:cluster{"Broadcasters":T4, "Receivers":T4})  [unwired: 1 in, 1 out]
              n120 = Unbundle By Name(w255) -> ("Receivers"=w257:T4)
              n121 = Insert Into Set(10:w256, 11:w257) -> (3:w254:T4)  [unwired: 1 out]
              n122 = Bundle By Name(cluster=w255, "Receivers"=w254) -> (w253:cluster{"Broadcasters":T4, "Receivers":T4})
              n123 = in-place-map #5(w253, LVMapReplaceAction."Add or Modify Entry" ("action")) -> (w250:T12)  [unwired: 2 out]
            }
          }
        }
        n124 = Bundle By Name(cluster=w241, "Actor View Map"=w237) -> (w238:T1)
      }
      frame "Publish To Actor View" {
        n125 = Unbundle By Name(w274) -> ("UI references.Actor View List"=w272:refnum<vi>, "Actor View Map"=w273:T13)
        n126 = for {
          tunnel: w273 -> [w277] mode=indexing
          tunnel: [w276] -> w271 mode=indexing
          n127 = Unbundle By Name(w277) -> ("Acor Name"=w276:string)
        }
        n128 = Build Array(w271) -> (w270:string[][])
        n129 = Transpose 2D Array(2D array=w270) -> (transposed array=w269:string[][])
        n130 = property class="MCListbox (strict)"(reference=w272, "ItemNames"=w269) -> ()  [unwired: 1 in, 2 out]
      }
      frame "Display Actor's Endpoints" {
        n131 = Unbundle By Name(w288) -> ("UI references.Actor View Broadcasters"=w284:refnum<vi>, "UI references.Actor View Receivers"=w282:refnum<vi>, "Actor View Map"=w287:T13, "MVA Project Path"=w279:path)
        n132 = Variant To Data(error in=w291, type="", Variant=w292) -> (data=w278:string, error out=w290:errorcluster)
        n133 = Look In Map(map=w287, key=w278) -> (value=w286:T11)  [unwired: 1 in, 1 out]
        n134 = Unbundle By Name(w286) -> ("Datum Broadcasters"=w285:T4, "Datum Receivers"=w283:T4)
        n135 = for {
          tunnel: w285 -> [w322] mode=indexing
          tunnel: [w314] -> w281 mode=indexing
          tunnel: w279 -> [w311]
          n136 = Unbundle By Name(w322) -> ("Datum Info.Datum Name"=w321:string, "Datum Info.Value is TypeDef"=w320:bool, "Datum Info.Type String"=w318:string, "Callng VI"=w310:path, "Source UID"=w313:i32, "Sink UID"=w312:i32)
          n137 = call <vilib>:"Compare Two Paths.vi"("Path 2"=w310, "Path 1"=w311) -> ("Relative Path from 1 to 2"=w309:path)  [unwired: 6 in, 3 out]
          n138 = Format Into String(w320) -> (resulting string=w319:string)  [unwired: 3 in, 1 out]
          n139 = Strip Path(path=w310) -> (name=w317:string)  [unwired: 1 out]
          n140 = Number To Decimal String(number=w313) -> (decimal integer string=w316:string)  [unwired: 1 in]
          n141 = Number To Decimal String(number=w312) -> (decimal integer string=w315:string)  [unwired: 1 in]
          n142 = Path To String(path=w309) -> (string=w308:string)
          n143 = Build Array(w321, w319, w318, w317, w316, w315, w308) -> (w314:string[])
        }
        n144 = for {
          tunnel: w283 -> [w307] mode=indexing
          tunnel: [w299] -> w280 mode=indexing
          tunnel: w279 -> [w295]
          n145 = Unbundle By Name(w307) -> ("Datum Info.Datum Name"=w306:string, "Datum Info.Value is TypeDef"=w305:bool, "Datum Info.Type String"=w303:string, "Callng VI"=w296:path, "Source UID"=w298:i32, "Sink UID"=w297:i32)
          n146 = Format Into String(w305) -> (resulting string=w304:string)  [unwired: 3 in, 1 out]
          n147 = call <vilib>:"Compare Two Paths.vi"("Path 2"=w296, "Path 1"=w295) -> ("Relative Path from 1 to 2"=w294:path)  [unwired: 6 in, 3 out]
          n148 = Strip Path(path=w296) -> (name=w302:string)  [unwired: 1 out]
          n149 = Number To Decimal String(number=w298) -> (decimal integer string=w301:string)  [unwired: 1 in]
          n150 = Number To Decimal String(number=w297) -> (decimal integer string=w300:string)  [unwired: 1 in]
          n151 = Path To String(path=w294) -> (string=w293:string)
          n152 = Build Array(w306, w304, w303, w302, w301, w300, w293) -> (w299:string[])
        }
        n153 = property class="MCListbox (strict)"(reference=w282, "ItemNames"=w280) -> ()  [unwired: 1 in, 2 out]
        n154 = property class="MCListbox (strict)"(reference=w284, "ItemNames"=w281) -> ()  [unwired: 1 in, 2 out]
      }
      frame "Display Data's End Points" {
        n155 = Variant To Data(error in=w339, type=0 ("NewVal"), Variant=w337) -> (data=w334:i32, error out=w338:errorcluster)
        n156 = Unbundle By Name(w335) -> ("UI references.Broadcasters"=w323:refnum<vi>, "UI references.Receivers"=w326:refnum<vi>, "MVA Project Path"=w327:path, "Message View Map"=w333:T2, "Message Map Keys"=w332:T3[])
        n157 = Index Array(array=w332, index=w334) -> (element=w331:T3)
        n158 = Look In Map(map=w333, key=w331) -> (value=w330:T11)  [unwired: 1 in, 1 out]
        n159 = Unbundle By Name(w330) -> ("Datum Broadcasters"=w329:T4, "Datum Receivers"=w328:T4)
        n160 = for {
          tunnel: w328 -> [w351] mode=indexing
          tunnel: w327 -> [w348]
          tunnel: [w344] -> w325 mode=indexing
          n161 = Unbundle By Name(w351) -> ("Callng VI"=w347:path, "Owning Class"=w349:string, "Source UID"=w343:i32, "Sink UID"=w341:i32)
          n162 = Number To Decimal String(number=w343) -> (decimal integer string=w342:string)  [unwired: 1 in]
          n163 = Strip Path(path=w347) -> (name=w350:string)  [unwired: 1 out]
          n164 = call <vilib>:"Compare Two Paths.vi"("Path 2"=w347, "Path 1"=w348) -> ("Relative Path from 1 to 2"=w346:path)  [unwired: 6 in, 3 out]
          n165 = Number To Decimal String(number=w341) -> (decimal integer string=w340:string)  [unwired: 1 in]
          n166 = Path To String(path=w346) -> (string=w345:string)
          n167 = Build Array(w350, w349, w345, w342, w340) -> (w344:string[])
        }
        n168 = for {
          tunnel: w329 -> [w363] mode=indexing
          tunnel: w327 -> [w360]
          tunnel: [w356] -> w324 mode=indexing
          n169 = Unbundle By Name(w363) -> ("Callng VI"=w359:path, "Owning Class"=w361:string, "Source UID"=w355:i32, "Sink UID"=w353:i32)
          n170 = Number To Decimal String(number=w353) -> (decimal integer string=w352:string)  [unwired: 1 in]
          n171 = Strip Path(path=w359) -> (name=w362:string)  [unwired: 1 out]
          n172 = call <vilib>:"Compare Two Paths.vi"("Path 2"=w359, "Path 1"=w360) -> ("Relative Path from 1 to 2"=w358:path)  [unwired: 6 in, 3 out]
          n173 = Number To Decimal String(number=w355) -> (decimal integer string=w354:string)  [unwired: 1 in]
          n174 = Path To String(path=w358) -> (string=w357:string)
          n175 = Build Array(w362, w361, w357, w354, w352) -> (w356:string[])
        }
        n176 = property class="MCListbox (strict)"(reference=w323, "ItemNames"=w324) -> ()  [unwired: 1 in, 2 out]
        n177 = property class="MCListbox (strict)"(reference=w326, "ItemNames"=w325) -> ()  [unwired: 1 in, 2 out]
      }
      frame "Open Block Diagram" {
        n178 = Variant To Data(error in=w384, type=T9 {"VI Name"="", "Owning Actor"="", "Sink UID"="", "Source UID"=""}, Variant=w385) -> (data=w370:T9)  [unwired: 1 out]
        n179 = Unbundle By Name(w383) -> ("MVA Project Reference"=w374:refnum<vi>)
        n180 = Unbundle By Name(w370) -> ("Owning Actor"=w368:string, "VI Name"=w369:string, "Source UID"=w367:string, "Sink UID"=w366:string)
        n181 = call <vilib>:"Split String.vi"("Ignore Case? (false)"=TRUE, "Split Pattern"=":", "Input String"=w368) -> ("Split String"=w377:string[])  [unwired: 4 in]
        n182 = Empty Array?(array=w377) -> (empty?=w376:bool)
        n183 = case shown="False" w376 {
          tunnel: w377 -> [w429 _]
          tunnel: [w428 w430] -> w372
          tunnel: [w426 _] -> w375
          tunnel: w368 -> [_ w430]
          frame False {
            n184 = Delete From Array(array=w429) -> (deleted portion=w428:string, array with subset deleted=w427:string[])  [unwired: 2 in]
            n185 = Reverse 1D Array(array=w427) -> (reversed array=w426:string[])
          }
          frame True {
          }
        }
        n186 = property class="Project"(reference=w374) -> ("Root"=w373:refnum<vi>)  [unwired: 1 in, 2 out]
        n187 = for {
          shift-right: [w435] -> w381
          shift-left: w373 -> [w436]
          tunnel: w375 -> [w431] mode=indexing
          shift-right: [w434] -> w380
          shift-left: _ -> [w433]
          tunnel: [w432] -> w365
          tunnel: [w431] -> w364
          stop <- w432 continue-if-true
          n188 = call <vilib>:"Get Proj Item Ref from Lib Name.vi"("ProjectItem in"=w436, "LIbrary Name"=w431, "error in (no error)"=w433) -> ("ProjectItem out"=w435:refnum<vi>, "Found"=w432:bool, "error out"=w434:errorcluster)  [unwired: 10 in]
        }
        n189 = case shown="False" w365 {
          tunnel: [_ w400] -> w382
          tunnel: w381 -> [_ w399]
          tunnel: w380 -> [_ w398]
          tunnel: w372 -> [_ w397]
          tunnel: w369 -> [_ w391]
          tunnel: w367 -> [_ w390]
          tunnel: w366 -> [_ w389]
          tunnel: w364 -> [w388 _]
          frame False {
            n190 = Format Into String(format string="This Library was not found under a project target. It may be in \ndependencies.\n%s", w388) -> (resulting string=w386:string)  [unwired: 2 in, 1 out]
            n191 = One Button Dialog(message=w386) -> ()  [unwired: 1 in, 1 out]
          }
          frame True {
            n192 = call <vilib>:"Get Proj Item Ref from Class Name.vi"("ProjectI tem"=w399, "Class Name"=w397, "error in (no error)"=w398) -> ("Class Project Item Reference"=w396:refnum<vi>, "error out"=w395:errorcluster)  [unwired: 10 in, 1 out]
            n193 = call <vilib>:"Get Proj Item Ref from VI Name.vi"("ProjectI tem"=w396, "VI Name"=w391, "error in (no error)"=w395) -> ("VI Project Item Reference"=w394:refnum<vi>, "Found"=w392:bool, "error out"=w393:errorcluster)  [unwired: 10 in]
            n194 = case shown="True" w392 {
              tunnel: [w401 w412] -> w400
              tunnel: w394 -> [_ w410]
              tunnel: w393 -> [w401 w409]
              tunnel: w390 -> [_ w403]
              tunnel: w389 -> [_ w402]
              frame False {
              }
              frame True {
                n195 = property class="ProjectItem"(reference=w410, error in=w409) -> (error out=w404:errorcluster, "Reference"=w408:refnum<vi>)  [unwired: 1 out]
                n196 = invoke class="VI" method="FP.Open"(reference=w408, error in=w404, "State"=T10."Minimized") -> (reference out=w421:refnum<vi>, error out=w419:errorcluster)  [unwired: 2 in, 3 out]
                n197 = property class="VI"(reference=w421, error in=w419, "BDWin.Open"=TRUE ("Block Diagram Window:Open")) -> (reference out=w418:refnum<vi>, error out=w417:errorcluster)
                n198 = Decimal String To Number(string=w402) -> (number=w411:i32)  [unwired: 2 in, 1 out]
                n199 = Decimal String To Number(string=w403) -> (number=w416:i32)  [unwired: 2 in, 1 out]
                n200 = call <vilib>:"UID to GObject Reference.vi"("error in (no error)"=w417, "UID"=w416, "Owning VI"=w418) -> ("error out"=w415:errorcluster, "GObject"=w407:refnum<vi>, "dup Owning VI"=w414:refnum<vi>)  [unwired: 6 in]
                n201 = call <vilib>:"UID to GObject Reference.vi"("error in (no error)"=w415, "UID"=w411, "Owning VI"=w414) -> ("error out"=w413:errorcluster, "GObject"=w405:refnum<vi>)  [unwired: 6 in, 1 out]
                n202 = Build Array(w407, w405) -> (w406:refnum<vi>[])
                n203 = for {
                  tunnel: w406 -> [w425] mode=indexing
                  shift-right: [w423] -> w412
                  shift-left: w413 -> [w424]
                  n204 = invoke class="GObj" method="ObjHighlight"(reference=w425, error in=w424) -> (error out=w423:errorcluster)  [unwired: 1 in, 2 out]
                }
              }
            }
          }
        }
      }
      frame "Navigate To VI" {
        n205 = Unbundle By Name(w446) -> ("MVA Project Reference"=w454:refnum<vi>)
        n206 = Variant To Data(type=T9 {"VI Name"="", "Owning Actor"="", "Sink UID"="", "Source UID"=""}, Variant=w455) -> (data=w448:T9)  [unwired: 1 in, 1 out]
        n207 = Unbundle By Name(w448) -> ("Owning Actor"=w447:string, "VI Name"=w445:string)
        n208 = property class="Project"(reference=w454) -> (error out=w443:errorcluster, "Root"=w444:refnum<vi>)  [unwired: 1 in, 1 out]
        n209 = call <vilib>:"Split String.vi"("Ignore Case? (false)"=TRUE, "Split Pattern"=":", "Input String"=w447) -> ("Split String"=w451:string[])  [unwired: 4 in]
        n210 = Empty Array?(array=w451) -> (empty?=w450:bool)
        n211 = case shown="False" w450 {
          tunnel: w451 -> [w477 _]
          tunnel: [w476 w489] -> w437
          tunnel: w447 -> [_ w489]
          tunnel: w444 -> [w474 w487]
          tunnel: w443 -> [w472 w488]
          tunnel: [w471 w487] -> w442
          tunnel: [w470 w488] -> w441
          frame False {
            # "Part of a library"
            n212 = Delete From Array(array=w477) -> (deleted portion=w476:string, array with subset deleted=w475:string[])  [unwired: 2 in]
            n213 = Reverse 1D Array(array=w475) -> (reversed array=w473:string[])
            n214 = for {
              shift-right: [w485] -> w471
              shift-left: w474 -> [w486]
              tunnel: w473 -> [w481] mode=indexing
              shift-right: [w484] -> w470
              shift-left: w472 -> [w483]
              tunnel: [w482] -> w468
              tunnel: [w481] -> w469
              stop <- w482 continue-if-true
              # "Navigate library hierarchy"
              n215 = call <vilib>:"Get Proj Item Ref from Lib Name.vi"("ProjectItem in"=w486, "LIbrary Name"=w481, "error in (no error)"=w483) -> ("ProjectItem out"=w485:refnum<vi>, "Found"=w482:bool, "error out"=w484:errorcluster)  [unwired: 10 in]
            }
            n216 = case shown="False" w468 {
              tunnel: w469 -> [w479 _]
              frame False {
                n217 = Format Into String(format string="This Library was not found under a project target. It may be in \ndependencies.\n%s", w479) -> (resulting string=w478:string)  [unwired: 2 in, 1 out]
                n218 = One Button Dialog(message=w478) -> ()  [unwired: 1 in, 1 out]
              }
              frame True {
              }
            }
          }
          frame True {
            # "Not a part of a library"
          }
        }
        n219 = call <vilib>:"Get Proj Item Ref from Class Name.vi"("ProjectI tem"=w442, "Class Name"=w437, "error in (no error)"=w441) -> ("Class Project Item Reference"=w440:refnum<vi>, "Found"=w438:bool, "error out"=w439:errorcluster)  [unwired: 10 in]
        n220 = case shown="True" w438 {
          tunnel: w445 -> [_ w464]
          tunnel: w440 -> [_ w463]
          tunnel: w439 -> [_ w460]
          tunnel: w437 -> [w457 _]
          frame False {
            n221 = Format Into String(format string="This Class was not found under a project target. It may be in \ndependencies.\n%s", w457) -> (resulting string=w458:string)  [unwired: 2 in, 1 out]
            n222 = One Button Dialog(message=w458) -> ()  [unwired: 1 in, 1 out]
          }
          frame True {
            n223 = call <vilib>:"Get Proj Item Ref from VI Name.vi"("ProjectI tem"=w463, "VI Name"=w464, "error in (no error)"=w460) -> ("VI Project Item Reference"=w462:refnum<vi>, "Found"=w461:bool)  [unwired: 10 in, 1 out]
            n224 = case shown="True" w461 {
              tunnel: w462 -> [_ w465]
              frame False {
              }
              frame True {
                n225 = invoke class="ProjectItem" method="SelectItem"(reference=w465, "Select"=TRUE, "ClearPreviousSelection"=TRUE) -> ()  [unwired: 2 in, 5 out]
              }
            }
          }
        }
      }
      frame "Navigate To Class" {
        n226 = Unbundle By Name(w505) -> ("MVA Project Reference"=w504:refnum<vi>)
        n227 = Variant To Data(type=T9 {"VI Name"="", "Owning Actor"="", "Sink UID"="", "Source UID"=""}, Variant=w506) -> (data=w500:T9)  [unwired: 1 in, 1 out]
        n228 = Unbundle By Name(w500) -> ("Owning Actor"=w498:string)
        n229 = call <vilib>:"Split String.vi"("Ignore Case? (false)"=TRUE, "Split Pattern"=":", "Input String"=w498) -> ("Split String"=w499:string[])  [unwired: 4 in]
        n230 = property class="Project"(reference=w504) -> (error out=w496:errorcluster, "Root"=w497:refnum<vi>)  [unwired: 1 in, 1 out]
        n231 = Empty Array?(array=w499) -> (empty?=w495:bool)
        n232 = case shown="False" w495 {
          tunnel: w499 -> [w523 _]
          tunnel: [w522 w535] -> w491
          tunnel: w498 -> [_ w535]
          tunnel: w497 -> [w520 w533]
          tunnel: w496 -> [w518 w534]
          tunnel: [w517 w533] -> w494
          tunnel: [w516 w534] -> w493
          frame False {
            # "Part of a library"
            n233 = Delete From Array(array=w523) -> (deleted portion=w522:string, array with subset deleted=w521:string[])  [unwired: 2 in]
            n234 = Reverse 1D Array(array=w521) -> (reversed array=w519:string[])
            n235 = for {
              shift-right: [w531] -> w517
              shift-left: w520 -> [w532]
              tunnel: w519 -> [w527] mode=indexing
              shift-right: [w530] -> w516
              shift-left: w518 -> [w529]
              tunnel: [w528] -> w514
              tunnel: [w527] -> w515
              stop <- w528 continue-if-true
              # "Navigate library hierarchy"
              n236 = call <vilib>:"Get Proj Item Ref from Lib Name.vi"("ProjectItem in"=w532, "LIbrary Name"=w527, "error in (no error)"=w529) -> ("ProjectItem out"=w531:refnum<vi>, "Found"=w528:bool, "error out"=w530:errorcluster)  [unwired: 10 in]
            }
            n237 = case shown="False" w514 {
              tunnel: w515 -> [w525 _]
              frame False {
                n238 = Format Into String(format string="This Library was not found under a project target. It may be in \ndependencies.\n%s", w525) -> (resulting string=w524:string)  [unwired: 2 in, 1 out]
                n239 = One Button Dialog(message=w524) -> ()  [unwired: 1 in, 1 out]
              }
              frame True {
              }
            }
          }
          frame True {
            # "Not a part of a library"
          }
        }
        n240 = call <vilib>:"Get Proj Item Ref from Class Name.vi"("ProjectI tem"=w494, "Class Name"=w491, "error in (no error)"=w493) -> ("Class Project Item Reference"=w490:refnum<vi>, "Found"=w492:bool)  [unwired: 10 in, 1 out]
        n241 = case shown="True" w492 {
          tunnel: w491 -> [w508 _]
          tunnel: w490 -> [_ w513]
          frame False {
            n242 = Format Into String(format string="This Class was not found under a project target. It may be in \ndependencies.\n%s", w508) -> (resulting string=w509:string)  [unwired: 2 in, 1 out]
            n243 = One Button Dialog(message=w509) -> ()  [unwired: 1 in, 1 out]
          }
          frame True {
            n244 = invoke class="ProjectItem" method="SelectItem"(reference=w513, "Select"=TRUE, "ClearPreviousSelection"=TRUE) -> ()  [unwired: 2 in, 5 out]
          }
        }
      }
      frame "Update Display" {
        # "Update Display - Convert the message data to a string to display in the Data Display indicator."
        n245 = Variant To Data(error in=w539, type="", Variant=w538) -> (error out=w536:errorcluster)  [unwired: 1 out]
        n246 = Merge Errors(w536) -> (w540:errorcluster)
      }
      frame "Error" {
        # "Error - Display an error dialog. This message is sent by the \"Error Handler\" VIs at the end of other loops in this application."
        n247 = Variant To Data(error in=w548, type=errorcluster {"status"=FALSE, "code"=0, "source"=""} ("error constant"), Variant=w546) -> (data=w544:errorcluster, error out=w543:errorcluster)
        n248 = Merge Errors(w543) -> (w542:errorcluster)
        n249 = call <vilib>:"Simple Error Handler.vi"("error in (no error)"=w544) -> ()  [unwired: 4 in, 5 out]
      }
      frame "Confirm Quit" {
        # "Confirm Quit - Message that can confirm whether or not the user wants to exit the application."
        n250 = call-poly <vilib>:"Enqueue Message.vi"("Priority Message? (F)"=TRUE, "error in (no error)"=w555, "Message"="Exit", "Message Queue"=w551) -> ("error out"=w552:errorcluster)  [unwired: 6 in, 1 out]
        n251 = Merge Errors(w552) -> (w553:errorcluster)
      }
      frame "---Copy This Frame---" {
        # "Duplicate this frame when creating new messages.  Change this comment in the duplicated frame to describe this message."
        n252 = Merge Errors(w558) -> (w556:errorcluster)
      }
      frame "Exit" {
        # "Exit - Exit the application."
        n253 = Variant To Data(type=errorcluster {"status"=FALSE, "code"=0, "source"=""} ("error constant"), Variant=w559) -> (data=w560:errorcluster)  [unwired: 1 in, 1 out]
        n254 = call <vilib>:"Fire User Event - Stop.vi"("User Event - Stop"=w564) -> ("error out"=w563:errorcluster)  [unwired: 10 in]
        n255 = Release Queue(queue=w569, error in (no error)=w562) -> (error out=w566:errorcluster)  [unwired: 1 in, 2 out]
        n256 = call <vilib>:"Simple Error Handler.vi"("error in (no error)"=w560) -> ()  [unwired: 4 in, 5 out]
        n257 = Merge Errors(w563, w566) -> (w565:errorcluster)
      }
      frame Default {
        # "'Default' case only runs if there is a message that isn't defined in any of the other cases.  Output a programming error."
        n258 = xnode "Error Ring"("parameter 0"=w570) -> ("error out"=w571:errorcluster)
      }
    }
    n259 = call <vilib>:"Error Handler - Message Handling Loop.vi"("error in (no error)"=w17, "Message Queue"=w19) -> ("dup error in"=w18:errorcluster)  [unwired: 8 in, 1 out]
  }
  n260 = while {
    tunnel: w13 -> [w588]
    shift-right: [w586] -> w9
    shift-left: w5 -> [w587]
    tunnel: [w582] -> w6
    shift-right: [w581] -> _
    shift-left: cluster{"Currently Selected Actor":string} {"Currently Selected Actor"=""} -> [w580]
    stop <- w584 stop-if-true
    # "Event Handling Loop"
    n261 = event shown="[10] \"Actor's Broadcasters\", \"Actor's Receivers\": Double Click" {
      selector: w587 -> [_ _ _ _ _ _ _ _ _ _ _ _]
      dyn-events: [_ _ _ _ _ _ _ _ _ _ _ _] -> w586
      timeout: _ -> [_ _ _ _ _ _ _ _ _ _ _ _]
      tunnel: [_ _ _ _ _ _ _ _ _ _ _ TRUE ("Discard?")] -> w584
      tunnel: w588 -> [w594 w597 w603 w608 w613 w618 w627 w647 w652 w663 w708 w743]
      tunnel: [w593 _ w602 w607 w611 _ _ _ w650 _ _ _] -> w585
      tunnel: [w592 w597 w601 w606 w612 w617 w622 w646 w651 w662 w707 w743] -> w583
      tunnel: [w589 w596 w598 w604 w609 w614 w619 w640 w648 w654 w701 w741] -> w581
      tunnel: w580 -> [w589 w596 w598 w604 w609 w614 w621 w640 w648 w654 w701 w741]
      event Panel Close? {
        n262 = event-data() -> ()  [unwired: 1 in, 1 out]
        n263 = call-poly <vilib>:"Enqueue Message.vi"("Priority Message? (F)"=TRUE, "Message"="Confirm Quit", "Message Queue"=w594) -> ("error out"=w593:errorcluster, "dup Message Queue"=w592:refnum<queue>)  [unwired: 7 in]
        n264 = event-data("Discard?"=TRUE) -> ()  [unwired: 1 in, 1 out]
      }
      event Application Instance Close {
        n265 = event-data() -> ()  [unwired: 1 in, 1 out]
      }
      event "Exit": Value Change {
        n266 = event-data() -> ()  [unwired: 1 in, 1 out]
        n267 = call-poly <vilib>:"Enqueue Message.vi"("Priority Message? (F)"=TRUE, "Message"="Exit", "Message Queue"=w603) -> ("error out"=w602:errorcluster, "dup Message Queue"=w601:refnum<queue>)  [unwired: 7 in]
      }
      event "Generate Cache": Value Change {
        n268 = event-data() -> ()  [unwired: 1 in, 1 out]
        n269 = call <vilib>:"Enqueue Message (Array).vi"("Message Array"=string[] ["Init Generate Cache", "Find Instances", "Populate Map"], "Message Queue"=w608) -> ("error out"=w607:errorcluster, "dup Message Queue"=w606:refnum<queue>)  [unwired: 8 in]
      }
      event "Load Cache": Value Change {
        n270 = event-data() -> ()  [unwired: 1 in, 1 out]
        n271 = call-poly <vilib>:"Enqueue Message.vi"("Message"="Check If Cache Exists", "Message Queue"=w613) -> ("error out"=w611:errorcluster, "dup Message Queue"=w612:refnum<queue>)  [unwired: 8 in]
      }
      event "Messages": Value Change {
        n272 = event-data() -> ("NewVal"=w615:i32)  [unwired: 1 in]
        n273 = call-poly <vilib>:"Enqueue Message.vi"("Message Data"=w615, "Message"="Display Data's End Points", "Message Queue"=w618) -> ("dup Message Queue"=w617:refnum<queue>)  [unwired: 7 in, 1 out]
      }
      event "Actor List": Value Change {
        n274 = event-data() -> ("CtlRef"=w626:refnum<vi>)  [unwired: 1 in]
        n275 = property class="MCListbox (strict)"(reference=w626) -> ("ItemNames"=w625:string[][])  [unwired: 1 in, 2 out]
        n276 = Index Array(array=w625, index (row)="Actor List", index (col)=0 ("disabled index (col)")) -> (element=w620:string)
        n277 = case shown="\"\"" w620 {
          selector: w620 -> [w631 _]
          tunnel: w627 -> [w634 w636]
          tunnel: [w632 w636] -> w622
          tunnel: w621 -> [w630 w635]
          tunnel: w620 -> [w629 _]
          tunnel: [w628 w635] -> w619
          frame Default {
            n278 = call-poly <vilib>:"Enqueue Message.vi"("Message Data"=w631, "Message"="Display Actor's Endpoints", "Message Queue"=w634) -> ("dup Message Queue"=w632:refnum<queue>)  [unwired: 7 in, 1 out]
            n279 = Bundle By Name(cluster=w630, "Currently Selected Actor"=w629) -> (w628:cluster{"Currently Selected Actor":string})
          }
          frame "" {
          }
        }
      }
      event "Actor List": Double Click {
        n280 = event-data() -> ("CtlRef"=w644:refnum<vi>)  [unwired: 1 in, 1 out]
        n281 = property class="MCListbox (strict)"(reference=w644) -> ("ItemNames"=w643:string[][], "Value"=w642:i32)  [unwired: 1 in, 2 out]
        n282 = Index Array(array=w643, index (row)=w642, index (col)=0 ("disabled index (col)")) -> (element=w638:string)
        n283 = Bundle By Name(cluster=T9 {"VI Name"="", "Owning Actor"="", "Sink UID"="", "Source UID"=""}, "Owning Actor"=w638) -> (w637:T9)
        n284 = call-poly <vilib>:"Enqueue Message.vi"("Message Data"=w637, "Message"="Navigate To Class", "Message Queue"=w647) -> ("dup Message Queue"=w646:refnum<queue>)  [unwired: 7 in, 1 out]
      }
      event "Cancel Generate": Value Change {
        n285 = event-data() -> ()  [unwired: 1 in, 1 out]
        n286 = call-poly <vilib>:"Enqueue Message.vi"("Priority Message? (F)"=TRUE, "Message"="Cancel Cache Generation", "Message Queue"=w652) -> ("error out"=w650:errorcluster, "dup Message Queue"=w651:refnum<queue>)  [unwired: 7 in]
      }
      event "Broadcasters", "Receivers": Double Click {
        n287 = event-data() -> ("CtlRef"=w661:refnum<vi>, "Row"=w660:i32, "Coords"=w658:T14)  [unwired: 1 in]
        n288 = property class="MCListbox (strict)"(reference=w661) -> (reference out=w659:refnum<vi>, "ItemNames"=w655:string[][])  [unwired: 1 in, 1 out]
        n289 = Index Array(array=w655, index (row)=w660) -> (element=w656:string[])  [unwired: 1 in]
        n290 = Empty Array?(array=w656) -> (empty?=w657:bool)
        n291 = case shown="False" w657 {
          tunnel: w663 -> [w672 w697]
          tunnel: [w671 w697] -> w662
          tunnel: w655 -> [w670 _]
          tunnel: w659 -> [w669 _]
          tunnel: w658 -> [w668 _]
          frame False {
            n292 = invoke class="MCListbox (strict)" method="Point To Row Column"(reference=w669, "Point"=w668) -> ("CellPosition"=w667:T15)  [unwired: 5 in, 6 out]
            n293 = Unbundle By Name(w667) -> ("Row"=w665:i32, "Column"=w666:i32)
            n294 = case shown="Default" w666 {
              selector: w666 -> [_ w691]
              tunnel: w672 -> [w687 w696]
              tunnel: [w686 w695] -> w671
              tunnel: w670 -> [w684 w693]
              tunnel: w665 -> [w677 w692]
              tunnel: T9 {"VI Name"="", "Owning Actor"="", "Sink UID"="", "Source UID"=""} -> [w680 w689]
              frame Default {
                n295 = Index Array(array=w684, index (row) #1=w677, index (col) #1=0 ("index"), index (row) #2=w677, index (col) #2=1 ("index"), index (row) #3=w677, index (col) #3=3 ("index"), index (row) #4=w677, index (col) #4=4 ("index")) -> (element #1=w679:string, element #2=w678:string, element #3=w675:string, element #4=w674:string)
                n296 = Bundle By Name(cluster=w680, "VI Name"=w679, "Owning Actor"=w678, "Sink UID"=w675, "Source UID"=w674) -> (w673:T9)
                n297 = call-poly <vilib>:"Enqueue Message.vi"("Message Data"=w673, "Message"="Open Block Diagram", "Message Queue"=w687) -> ("dup Message Queue"=w686:refnum<queue>)  [unwired: 7 in, 1 out]
              }
              frame 1 {
                n298 = Index Array(array=w693, index (row)=w692, index (col)=w691) -> (element=w690:string)
                n299 = Bundle By Name(cluster=w689, "Owning Actor"=w690) -> (w688:T9)
                n300 = call-poly <vilib>:"Enqueue Message.vi"("Message Data"=w688, "Message"="Navigate To Class", "Message Queue"=w696) -> ("dup Message Queue"=w695:refnum<queue>)  [unwired: 7 in, 1 out]
              }
            }
          }
          frame True {
          }
        }
      }
      event "Actor's Broadcasters", "Actor's Receivers": Double Click {
        n301 = event-data() -> ("CtlRef"=w706:refnum<vi>, "Row"=w705:i32, "Coords"=w699:T14)  [unwired: 1 in]
        n302 = Unbundle By Name(w701) -> ("Currently Selected Actor"=w700:string)
        n303 = property class="MCListbox (strict)"(reference=w706) -> (reference out=w704:refnum<vi>, "ItemNames"=w698:string[][])  [unwired: 1 in, 1 out]
        n304 = Index Array(array=w698, index (row)=w705) -> (element=w702:string[])  [unwired: 1 in]
        n305 = Empty Array?(array=w702) -> (empty?=w703:bool)
        n306 = case shown="False" w703 {
          tunnel: w708 -> [w718 w740]
          tunnel: [w717 w740] -> w707
          tunnel: w702 -> [w716 _]
          tunnel: w704 -> [w714 _]
          tunnel: w700 -> [w715 _]
          tunnel: w699 -> [w713 _]
          tunnel: w698 -> [w709 _]
          frame False {
            n307 = invoke class="MCListbox (strict)" method="Point To Row Column"(reference=w714, "Point"=w713) -> ("CellPosition"=w712:T15)  [unwired: 5 in, 6 out]
            n308 = Unbundle By Name(w712) -> ("Row"=w710:i32, "Column"=w711:i32)
            n309 = case shown="3" w711 {
              tunnel: w718 -> [w729 w739]
              tunnel: [w728 w738] -> w717
              tunnel: w716 -> [w726 _]
              tunnel: w715 -> [w719 w734]
              tunnel: w710 -> [_ w732]
              tunnel: w709 -> [_ w733]
              frame Default {
                n310 = Index Array(array=w726, index #1=3 ("index")) -> (element #1=w721:string, element #2=w724:string, element #3=w723:string)  [unwired: 2 in]
                n311 = Bundle By Name(cluster=T9 {"VI Name"="", "Owning Actor"="", "Sink UID"="", "Source UID"=""}, "Owning Actor"=w719, "VI Name"=w721, "Source UID"=w724, "Sink UID"=w723) -> (w722:T9)
                n312 = call-poly <vilib>:"Enqueue Message.vi"("Message Data"=w722, "Message"="Open Block Diagram", "Message Queue"=w729) -> ("dup Message Queue"=w728:refnum<queue>)  [unwired: 7 in, 1 out]
              }
              frame 3 {
                n313 = Index Array(array=w733, index (row)=w732, index (col)=3 ("disabled index (col)")) -> (element=w731:string)
                n314 = Bundle By Name(cluster=T9 {"VI Name"="", "Owning Actor"="", "Sink UID"="", "Source UID"=""}, "Owning Actor"=w734, "VI Name"=w731) -> (w735:T9)
                n315 = call-poly <vilib>:"Enqueue Message.vi"("Message Data"=w735, "Message"="Navigate To VI", "Message Queue"=w739) -> ("dup Message Queue"=w738:refnum<queue>)  [unwired: 7 in, 1 out]
              }
            }
          }
          frame True {
          }
        }
      }
      event User Event {
        n316 = event-data() -> ()  [unwired: 1 in, 1 out]
      }
    }
    n317 = call <vilib>:"Error Handler - Event Handling Loop.vi"("error in (no error)"=w585, "Message Queue"=w583) -> ("dup error in"=w582:errorcluster)  [unwired: 8 in, 1 out]
  }
  n318 = Unregister For Events(event registration refnum=w9, error in=w6) -> (error out=w10:errorcluster)
  n319 = Merge Errors(w10, w14) -> (w11:errorcluster)
  n320 = call <vilib>:"Destroy User Event - Stop.vi"("error in (no error)"=w11, "User Event - Stop"=w4) -> ("error out"=w7:errorcluster)  [unwired: 9 in]
  n321 = disable-structure "Conditional Disable Structure" shown="RUN_TIME_ENGINE==True" {
    disable-tunnel: w7 -> [_ _]
    frame condition #0 (active) {
    }
    frame condition #1 {
      # "Call Quit LabVIEW if running as a built application."
      n322 = Quit LabVIEW() -> ()  [unwired: 1 in]
    }
  }
